vi "Draw Frame.vi"(8 "Error In":errorcluster, 11 "Draw Frame In":refnum<class "Draw Frame.lvclass">) -> (0 "Error Out":errorcluster, 3 "Draw Frame Out":refnum<class "Draw Frame.lvclass">)   [LabVIEW 2021, in "Draw Frame.lvclass"]
uses:
  Draw Frame.lvclass
  Accessors/Display/Get Display.vi
  <vilib>/Memosfet/myRIO-Neopixel/RT/Display/Display.lvclass
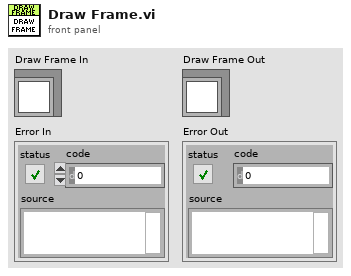
[diagram p1: front panel]
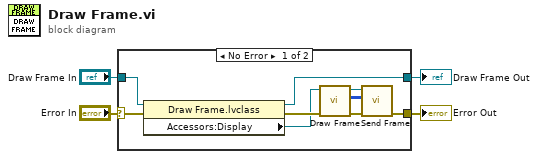
[diagram p0: block diagram]
diagram:
  n1 = case shown="No Error" "Error In" {
    selector: "Error In" -> [w11 w14]
    tunnel: [w5 w14] -> w4
    tunnel: "Draw Frame In" -> [w13 w15]
    tunnel: [w12 w15] -> w2
    frame No Error {
      n2 = property class="Draw Frame.lvclass"(reference=w13, error in=w11) -> (reference out=w12:refnum<class "Draw Frame.lvclass">, error out=w10:errorcluster, "Accessors:Display"=w9:refnum<class "Display.lvclass">)
      n3 = call <vilib>:"Draw Frame.vi"("Error In"=w10, "Display In"=w9) -> ("Error Out"=w6:errorcluster, "Frame"=w7:u32[][], "Display Out"=w8:refnum<class "Display.lvclass">)  [unwired: 7 in]
      n4 = call <vilib>:"Send Frame.vi"("Error In"=w6, "Frame"=w7, "Display In"=w8) -> ("Error Out"=w5:errorcluster)  [unwired: 7 in, 1 out]
    }
    frame Error {
    }
  }
  "Error Out" <- w4
  "Draw Frame Out" <- w2
